vi "SendPbAddr.vi"(7 "error in (no error)":errorcluster, 9 "PICOBUS ADDRESS":u8=1 min=1 max=15 step=1, 10 "VISA resource":refnum<visa-resource-name>="COM1") -> (0 "error out":errorcluster, 3 "dup VISA resource":refnum<visa-resource-name>="COM1")   [LabVIEW 2023]
doc: "Sends address string\nto AVS-47B"
panel:
  # "Send Picobus Address (PBA) v2.0"
  # "SendPbAddr.vi"
  # "Sends the Picobus Address (PBA) to the AVS-47B. All Picobus transactions with\n the bridge consist of the following sequence:\n\n1) send Picobus address (8 bits)\n2) strobe the address\n3) send and read data (48 bits)\n4) strobe the data\n\nEvery transaction contains both writing (a possibly new) configuration and \nreading the existing (old) configuration from the bridge. Together with the \nconfiguration, the AVS-47B sends also the result of the latest A/D conversion to the PC.  \nReading the conversion result does not reset it."
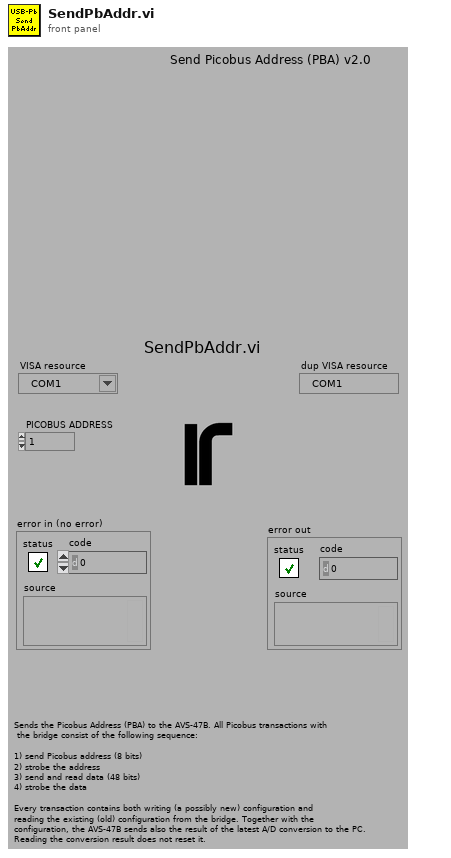
[diagram p1: front panel]
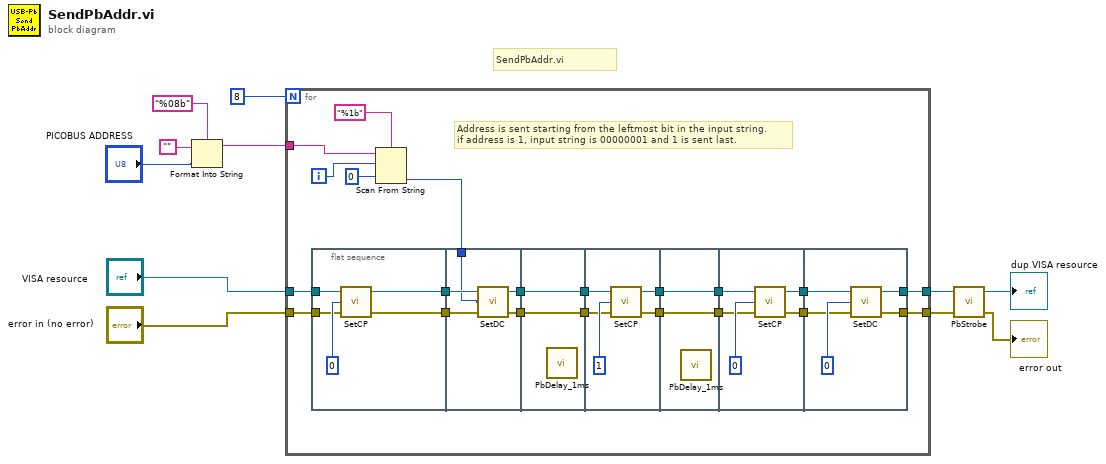
[diagram p0: block diagram]
diagram:
  # "SendPbAddr.vi"
  n1 = Format Into String(format string="%08b", initial string="", "PICOBUS ADDRESS") -> (resulting string=w8:string)  [unwired: 1 in, 1 out]
  n2 = for {
    N: 8 -> [_]
    tunnel: w8 -> [w32]
    tunnel: "error in (no error)" -> [w16]
    tunnel: "VISA resource" -> [w15]
    tunnel: [w14] -> w5
    tunnel: [w13] -> w4
    i -> [w31]
    # "Address is sent starting from the leftmost bit in the input string.\nif address is 1, input string is 00000001 and 1 is sent last."
    n3 = flat-sequence {
      tunnel: w15 -> [w37]
      tunnel: [w36] -> w28
      tunnel: w16 -> [w34]
      tunnel: [w33] -> w27
      tunnel: w28 -> [w42]
      tunnel: [w41] -> w26
      tunnel: w27 -> [w40]
      tunnel: [w39] -> w25
      tunnel: w12 -> [w38]
      tunnel: [w44] -> w24
      tunnel: w26 -> [w44]
      tunnel: [w43] -> w23
      tunnel: w25 -> [w43]
      tunnel: w24 -> [w49]
      tunnel: [w48] -> w22
      tunnel: w23 -> [w46]
      tunnel: [w45] -> w21
      tunnel: [w51] -> w20
      tunnel: w22 -> [w51]
      tunnel: [w50] -> w19
      tunnel: w21 -> [w50]
      tunnel: w20 -> [w56]
      tunnel: [w55] -> w18
      tunnel: w19 -> [w53]
      tunnel: [w52] -> w17
      tunnel: w18 -> [w61]
      tunnel: w17 -> [w59]
      tunnel: [w58] -> w13
      tunnel: [w57] -> w14
      frame #0 {
        n4 = call "SetCP.vi"("error in (no error)"=w34, "CP(=RTS) state"=u8 0, "VISA resource"=w37) -> ("error out"=w33:errorcluster, "dup VISA resource"=w36:refnum<visa-resource-name>)  [unwired: 1 in]
      }
      frame #1 {
        n5 = call "SetDC.vi"("error in (no error)"=w40, "DC(=DTR) state"=w38, "VISA resource"=w42) -> ("error out"=w39:errorcluster, "dup VISA resource"=w41:refnum<visa-resource-name>)  [unwired: 1 in]
      }
      frame #2 {
        n6 = call "PbDelay_1ms.vi"() -> ()  [unwired: 4 in]
      }
      frame #3 {
        n7 = call "SetCP.vi"("error in (no error)"=w46, "CP(=RTS) state"=u8 1, "VISA resource"=w49) -> ("error out"=w45:errorcluster, "dup VISA resource"=w48:refnum<visa-resource-name>)  [unwired: 1 in]
      }
      frame #4 {
        n8 = call "PbDelay_1ms.vi"() -> ()  [unwired: 4 in]
      }
      frame #5 {
        n9 = call "SetCP.vi"("error in (no error)"=w53, "CP(=RTS) state"=u8 0, "VISA resource"=w56) -> ("error out"=w52:errorcluster, "dup VISA resource"=w55:refnum<visa-resource-name>)  [unwired: 1 in]
      }
      frame #6 {
        n10 = call "SetDC.vi"("error in (no error)"=w59, "DC(=DTR) state"=u8 0, "VISA resource"=w61) -> ("error out"=w58:errorcluster, "dup VISA resource"=w57:refnum<visa-resource-name>)  [unwired: 1 in]
      }
    }
    n11 = Scan From String(format string="%1b", input string=w32, initial scan location=w31, default 1=u8 0) -> (output 1=w12:u8)  [unwired: 1 in, 3 out]
  }
  n12 = call "PbStrobe.vi"("error in (no error)"=w4, "VISA resource"=w5) -> ("error out"=→"error out":errorcluster, "dup VISA resource"=→"dup VISA resource":refnum<visa-resource-name>)  [unwired: 2 in]
